vi "Config GUI - Init.vi"(8 "Error In":errorcluster, 11 "VI Reference":refnum<vi>) -> (0 "Error Out":errorcluster)   [LabVIEW 2023, in "Error Manager.lvlib" / "Anti-Spam Tester (AST).lvlib"]
doc: "Blank VI with error handling."
uses:
  Anti-Spam Tester (AST).lvlib
panel:
  # "Input\nInputs to the VI"
  # "Development\nControls or indicators that are useful for development or testing, but which are not outputs of the VI."
  # "Output\nOutputs of the VI"
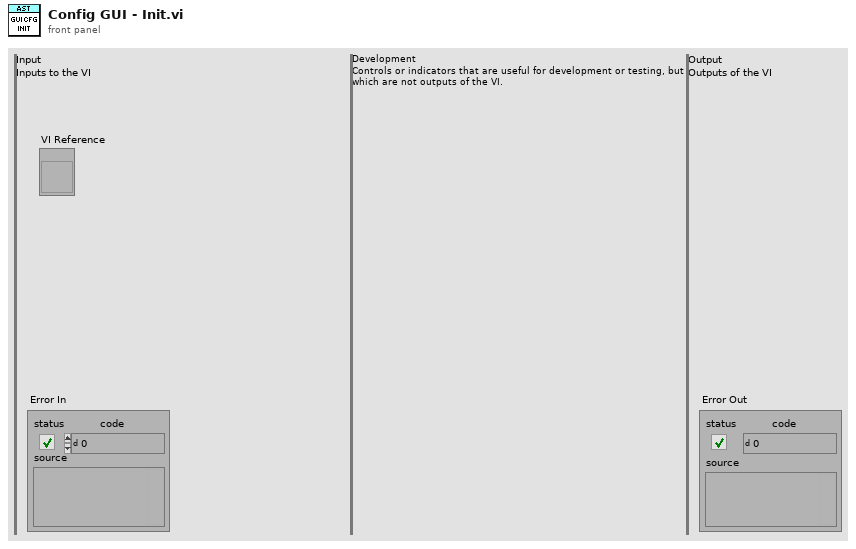
[diagram p1: front panel]
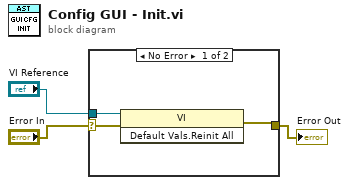
[diagram p0: block diagram]
diagram:
  n1 = case shown="No Error" "Error In" {
    selector: "Error In" -> [w6 w7]
    tunnel: [w5 w7] -> w2
    tunnel: "VI Reference" -> [w4 _]
    frame No Error {
      n2 = invoke class="VI" method="Default Vals.Reinit All"(reference=w4, error in=w6) -> (error out=w5:errorcluster)  [unwired: 1 in, 2 out]
    }
    frame Error {
    }
  }
  "Error Out" <- w2
